vi "HDF5_Init_AI_Refs.vi"(5 "HDF5 file ref":T1 format="%.0x", 9 "File Exists?":bool, 11 "error in":errorcluster) -> (4 "AI_Refs":T2 {"BlowerPwr_dset" format="%.0x"; "ElStdDev_dset" format="%.0x"; "AzStdDev_dset" format="%.0x"; "AI19_dset" format="%.0x"; "AI18_dset" format="%.0x"; "AI17_dset" format="%.0x"; "AI16_dset" format="%.0x"; "AI6_dset" format="%.0x"; "AI5_dset" format="%.0x"; "AI4_dset" format="%.0x"; "AI3_dset" format="%.0x"; "AI2_dset" format="%.0x"; "AI0_dset" format="%.0x"; "AI1_dset" format="%.0x"; "TimeString_dset" format="%.0x"; "TimeStamp_dset" format="%.0x"; "Group_ref" format="%.0x"}, 15 "error out":errorcluster)   [LabVIEW 2018]
doc: "Set up the HDF5 data structure and initialize the references for the AI Datasets (tables).\n\nData structure:\nAI (Dataset) - 16 element Double array (waveform) x 100,000 records"
uses:
  HDF5_AI_refs.ctl
  <vilib>/addons/h5labview2/base/hid_t.ctl
  lib_path_mod_20200519.vi
  <vilib>/addons/h5labview2/base/H5Equery.vi
  <vilib>/addons/h5labview2/attrib/H5Awrite.llb/H5Awrite.xnode
  <vilib>/addons/h5labview2/group/H5G.lvlib
  <vilib>/addons/h5labview2/dataset/H5D.lvlib
panel:
  out "HDF5 file ref 3":T1 format="%.0x"
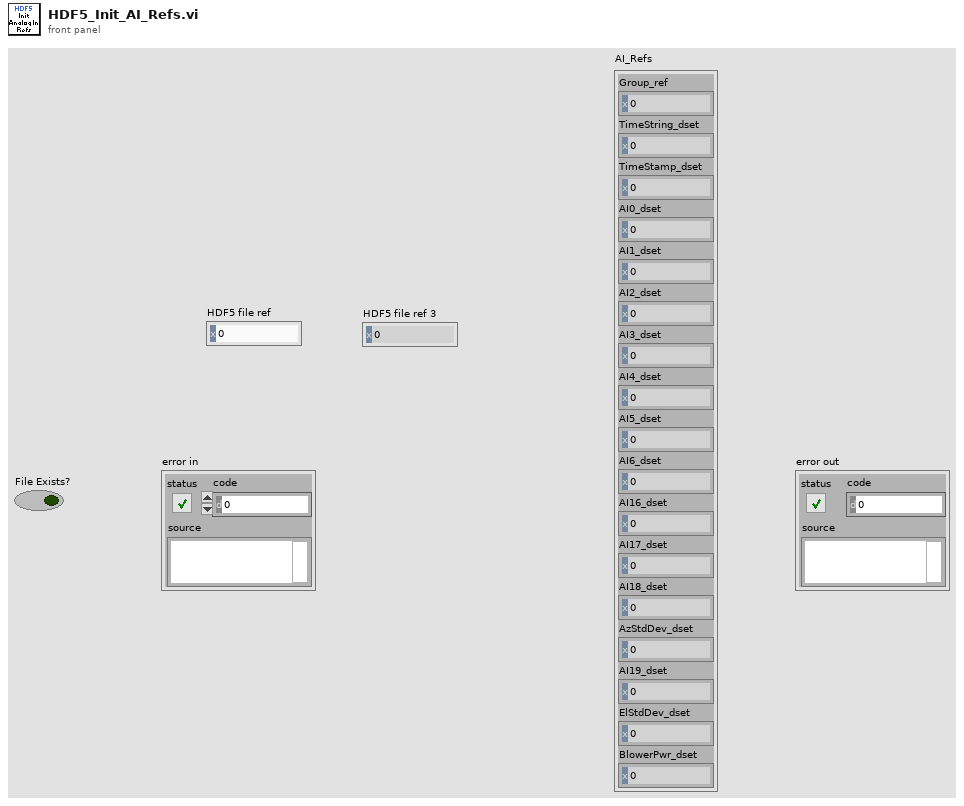
[diagram p1: front panel]
types:
  T1 = typedef "hid_t.ctl" = i32
  T2 = typedef "HDF5_AI_refs.ctl" = cluster{"Group_ref":T1, "TimeString_dset":T1, "TimeStamp_dset":T1, "AI0_dset":T1, "AI1_dset":T1, "AI2_dset":T1, "AI3_dset":T1, "AI4_dset":T1, "AI5_dset":T1, "AI6_dset":T1, "AI16_dset":T1, "AI17_dset":T1, "AI18_dset":T1, "AzStdDev_dset":T1, "AI19_dset":T1, "ElStdDev_dset":T1, "BlowerPwr_dset":T1}
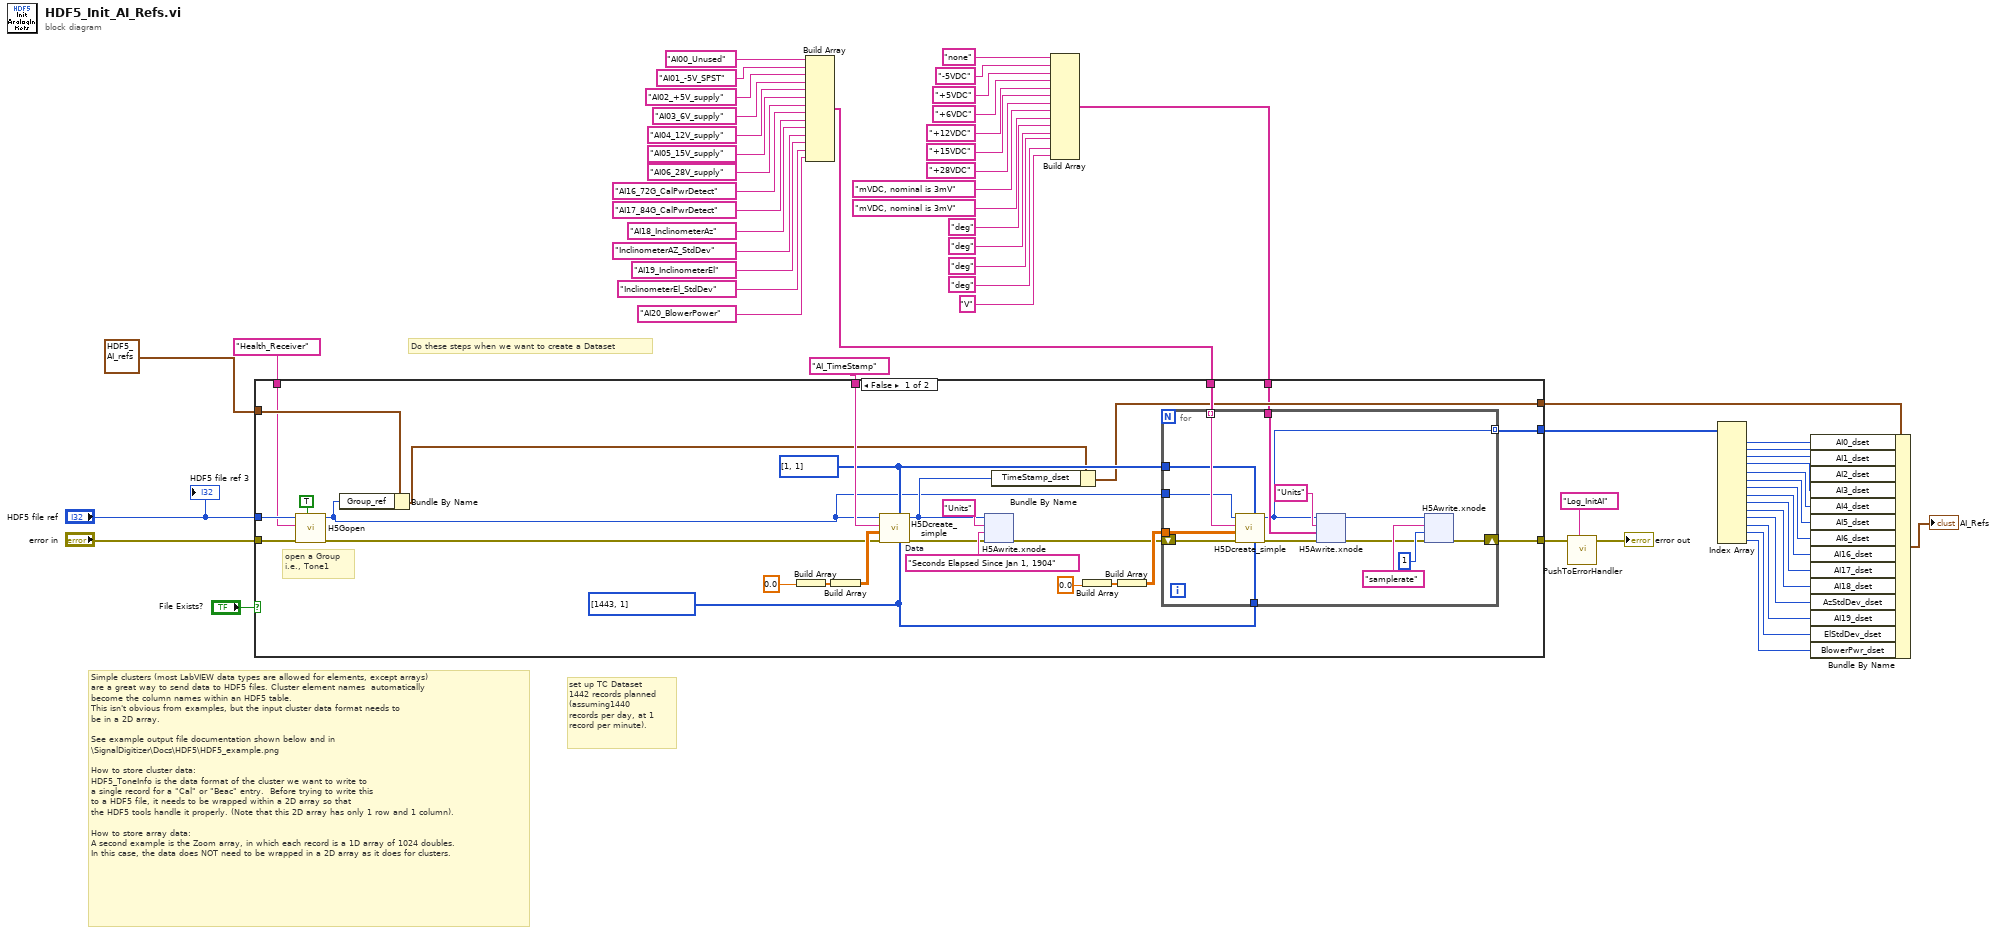
[diagram p0: block diagram]
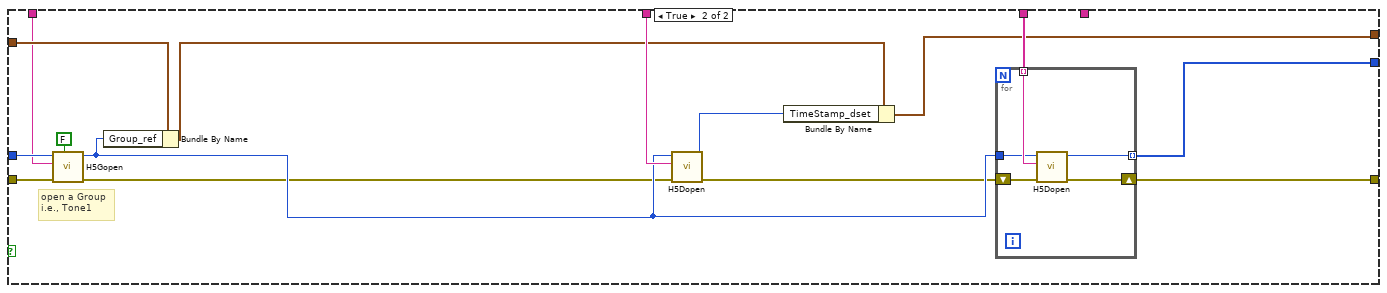
[diagram p2: hidden frame]
diagram:
  # "Do these steps when we want to create a Dataset"
  # "set up TC Dataset\n1442 records planned\n(assuming1440\nrecords per day, at 1\nrecord per minute)."
  # "Simple clusters (most LabVIEW data types are allowed for elements, except arrays) \nare a great way to send data to HDF5 files. Cluster element names  automatically\nbecome the column names within an HDF5 table.\nThis isn't obvious from examples, but the input cluster data format needs to \nbe in a 2D array.\n\nSee example output file documentation shown below and in\n\\SignalDigitizer\\Docs\\HDF5\\HDF5_example.png\n\nHow to store cluster data:\nHDF5_ToneInfo is the data format of the cluster we want to write to \na single record for a \"Cal\" or \"Beac\" entry.  Before trying to write this \nto a HDF5 file, it needs to be wrapped within a 2D array so that \nthe HDF5 tools handle it properly. (Note that this 2D array has only 1 row and 1 column).\n\nHow to store array data:\nA second example is the Zoom array, in which each record is a 1D array of 1024 doubles.\nIn this case, the data does NOT need to be wrapped in a 2D array as it does for clusters."
  n1 = Build Array("AI00_Unused" ("string"), "AI01_-5V_SPST" ("string"), "AI02_+5V_supply" ("string"), "AI03_6V_supply" ("string"), "AI04_12V_supply" ("string"), "AI05_15V_supply" ("string"), "AI06_28V_supply" ("string"), "AI16_72G_CalPwrDetect" ("string"), "AI17_84G_CalPwrDetect" ("string"), "AI18_InclinometerAz" ("string"), "InclinometerAZ_StdDev" ("string"), "AI19_InclinometerEl" ("string"), "InclinometerEl_StdDev" ("string"), "AI20_BlowerPower" ("string")) -> (w32:string[])
  n2 = Build Array("none" ("string"), "-5VDC" ("string"), "+5VDC" ("string"), "+6VDC" ("string"), "+12VDC" ("string"), "+15VDC" ("string"), "+28VDC" ("string"), "mVDC, nominal is 3mV" ("string"), "mVDC, nominal is 3mV" ("string"), "deg" ("string"), "deg" ("string"), "deg" ("string"), "deg" ("string"), "V" ("string")) -> (w22:string[])
  n3 = case shown="False" "File Exists?" {
    tunnel: "error in" -> [w83 w170]
    tunnel: "HDF5 file ref" -> [w82 w169]
    tunnel: [w68 w161] -> w18
    tunnel: T2 {"Group_ref"=0, "TimeString_dset"=0, "TimeStamp_dset"=0, "AI0_dset"=0, "AI1_dset"=0, "AI2_dset"=0, "AI3_dset"=0, "AI4_dset"=0, "AI5_dset"=0, "AI6_dset"=0, "AI16_dset"=0, "AI17_dset"=0, "AI18_dset"=0, "AzStdDev_dset"=0, "AI19_dset"=0, "ElStdDev_dset"=0, "BlowerPwr_dset"=0} ("Cluster") -> [w80 w167]
    tunnel: "AI_TimeStamp" ("string") -> [w79 w166]
    tunnel: w32 -> [w76 w164]
    tunnel: [w70 w160] -> w42
    tunnel: [w69 w159] -> w40
    tunnel: w22 -> [w63 _]
    tunnel: "Health_Receiver" ("name") -> [w61 w158]
    frame False {
      w58 = u64[] [1443, 1] ("max size")
      w67 = "Seconds Elapsed Since Jan 1, 1904"  # Data
      w71 = u64[] [1, 1] ("chunk size")
      # "open a Group\ni.e., Tone1"
      n4 = call <vilib>:"H5Gopen.vi"("create? (F)"=TRUE, "error in (no error)"=w83, "name"=w61, "ref in"=w82) -> ("error out"=w59:errorcluster, "group out"=w57:T1)  [unwired: 6 in]
      n5 = Bundle By Name(cluster=w80, "Group_ref"=w57) -> (w60:T2)
      n6 = Build Array(0.0 ("TimeStamp")) -> (w77:dbl[])
      n7 = Build Array(w77) -> (w78:dbl[][])
      n8 = call <vilib>:"H5Dcreate_simple.vi"("max size"=w58, "chunk size"=w71, "error in (no error)"=w59, "type in"=w78, "name"=w79, "ref in"=w57) -> ("error out"=w65:errorcluster, "dset out"=w62:T1)  [unwired: 4 in]
      n9 = xnode "H5Awrite.xnode"("error in (no error)"=w65, "data"=w67, "attrib name"="Units", "ref in"=w62) -> ("error out"=w64:errorcluster)  [unwired: 3 in, 2 out]
      n10 = Bundle By Name(cluster=w60, "TimeStamp_dset"=w62) -> (w70:T2)
      n11 = Build Array(0.0) -> (w74:dbl[])
      n12 = Build Array(w74) -> (w75:dbl[][])
      n13 = for {
        tunnel: w76 -> [w117] mode=indexing
        tunnel: w75 -> [w116]
        tunnel: w58 -> [w114]
        tunnel: w71 -> [w113]
        tunnel: w57 -> [w112]
        tunnel: [w108] -> w69 mode=indexing
        shift-right: [w104] -> w68
        shift-left: w64 -> [w115]
        tunnel: w63 -> [w109]
        n14 = call <vilib>:"H5Dcreate_simple.vi"("max size"=w114, "chunk size"=w113, "error in (no error)"=w115, "type in"=w116, "name"=w117, "ref in"=w112) -> ("error out"=w110:errorcluster, "dset out"=w108:T1)  [unwired: 4 in]
        n15 = xnode "H5Awrite.xnode"("error in (no error)"=w110, "data"=w109, "attrib name"="Units", "ref in"=w108) -> ("error out"=w105:errorcluster, "ref out"=w103:i32)  [unwired: 3 in, 1 out]
        n16 = xnode "H5Awrite.xnode"("error in (no error)"=w105, "data"=u32 1, "attrib name"="samplerate", "ref in"=w103) -> ("error out"=w104:errorcluster)  [unwired: 3 in, 2 out]
      }
    }
    frame True {
      # "open a Group\ni.e., Tone1"
      n17 = call <vilib>:"H5Gopen.vi"("create? (F)"=FALSE, "error in (no error)"=w170, "name"=w158, "ref in"=w169) -> ("error out"=w156:errorcluster, "group out"=w163:T1)  [unwired: 6 in]
      n18 = Bundle By Name(cluster=w167, "Group_ref"=w163) -> (w157:T2)
      n19 = call <vilib>:"H5Dopen.vi"("error in (no error)"=w156, "name"=w166, "loc in"=w163) -> ("error out"=w162:errorcluster, "dset out"=w165:T1)  [unwired: 7 in]
      n20 = Bundle By Name(cluster=w157, "TimeStamp_dset"=w165) -> (w160:T2)
      n21 = for {
        tunnel: w164 -> [w175] mode=indexing
        tunnel: w163 -> [w174]
        shift-right: [w172] -> w161
        shift-left: w162 -> [w173]
        tunnel: [w171] -> w159 mode=indexing
        n22 = call <vilib>:"H5Dopen.vi"("error in (no error)"=w173, "name"=w175, "loc in"=w174) -> ("error out"=w172:errorcluster, "dset out"=w171:T1)  [unwired: 7 in]
      }
    }
  }
  n23 = call "PushToErrorHandler.vi"("ErrorIn"=w18, "ErrorLocation"="Log_InitAI") -> ("ErrorOut"=→"error out":errorcluster)  [unwired: 5 in]
  n24 = Index Array(array=w40) -> (element #1=w39:T1, element #2=w38:T1, element #3=w37:T1, element #4=w36:T1, element #5=w35:T1, element #6=w34:T1, element #7=w33:T1, element #8=w21:T1, element #9=w20:T1, element #10=w11:T1, element #11=w4:T1, element #12=w6:T1, element #13=w5:T1, element #14=w1:T1)  [unwired: 14 in]
  n25 = Bundle By Name(cluster=w42, "AI0_dset"=w39, "AI1_dset"=w38, "AI2_dset"=w37, "AI3_dset"=w36, "AI4_dset"=w35, "AI5_dset"=w34, "AI6_dset"=w33, "AI16_dset"=w21, "AI17_dset"=w20, "AI18_dset"=w11, "AzStdDev_dset"=w4, "AI19_dset"=w6, "ElStdDev_dset"=w5, "BlowerPwr_dset"=w1) -> (→"AI_Refs":T2)
  "HDF5 file ref 3" <- "HDF5 file ref"
